vi "SNR formula_modified for Express.vi"(1 "THD [ratio]":dbl=1e-06 format="%.2e", 2 "SINAD [dB]":dbl=118.0 format="%.2p") -> (0 "SNR [dB]":dbl=122.32923433336248)   [LabVIEW 2017]
panel:
  # "This subVI assumes that the SINAD and THD inputs are in the units returned by the Distortion Express VI. \nDo not modify the distortion VI outputs before wiring them to this subVI."
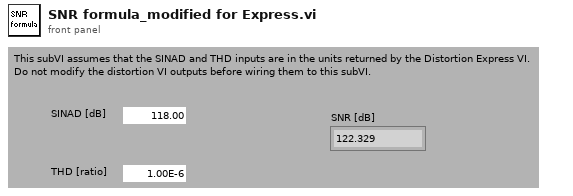
[diagram p1: front panel]
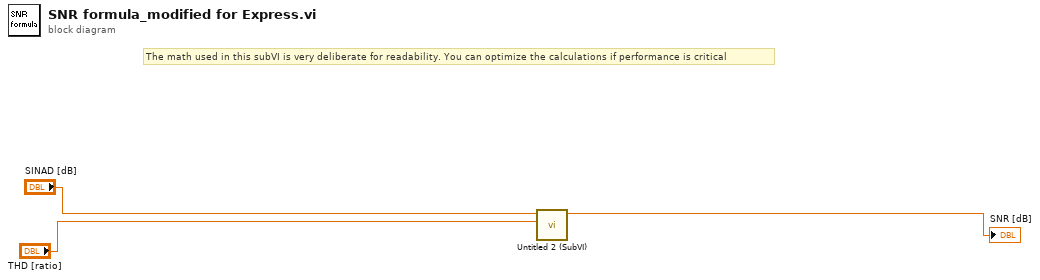
[diagram p0: block diagram]
diagram:
  # "The math used in this subVI is very deliberate for readability. You can optimize the calculations if performance is critical"
  n1 = call "Untitled 2 (SubVI).vi"("THD [ratio]"="THD [ratio]", "SINAD [dB]"="SINAD [dB]") -> ("dBSNR"=→"SNR [dB]":dbl)  [unwired: 9 in]
